vi "Linear Regression Code.vi"(7 "Ordered Pairs":T1, 10 "Number of Pairs":i32) -> (0 "Slope Angle":dbl, 3 "Intercept":dbl)   [LabVIEW 2012]
uses:
  <vilib>/Analysis/Matrix/Datatypes/RealMatrix.ctl
  <vilib>/Analysis/Matrix/NI_Matrix.lvlib
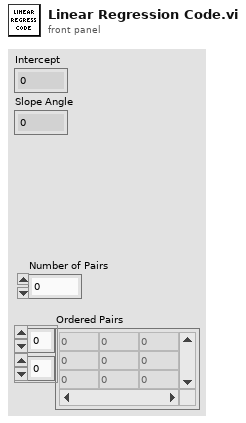
[diagram p1: front panel]
types:
  T1 = typedef "NI_Matrix.lvlib/RealMatrix.ctl" = dbl[][]
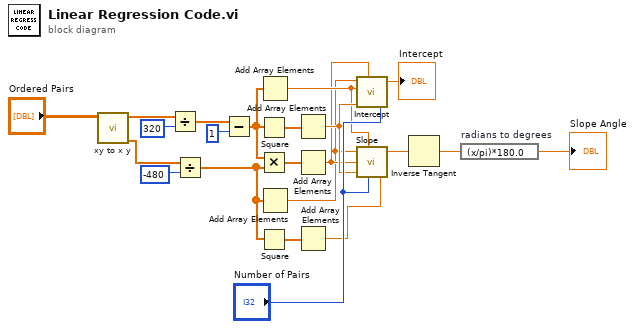
[diagram p0: block diagram]
diagram:
  n1 = call "xy to x y.vi"("Ordered Pairs"="Ordered Pairs") -> ("Y"=w1:dbl[], "X"=w2:dbl[])  [unwired: 9 in]
  n2 = Divide(x=w2, y=320) -> (x/y=w21:dbl[])
  n3 = Divide(x=w1, y=-480) -> (x/y=w15:dbl[])
  n4 = Subtract(x=w21, y=1) -> (x-y=w17:dbl[])
  n5 = Square(x=w17) -> (x^2=w16:dbl[])
  n6 = Multiply(x=w17, y=w15) -> (x*y=w18:dbl[])
  n7 = Square(x=w15) -> (x^2=w14:dbl[])
  n8 = Add Array Elements(numeric array=w17) -> (sum=w11:dbl)
  n9 = Add Array Elements(numeric array=w15) -> (sum=w9:dbl)
  n10 = Add Array Elements(numeric array=w16) -> (sum=w12:dbl)
  n11 = Add Array Elements(numeric array=w18) -> (sum=w10:dbl)
  n12 = Add Array Elements(numeric array=w14) -> (sum=w6:dbl)
  n13 = call "Intercept.vi"("Y"=w9, "X"=w11, "X2"=w12, "XY"=w10, "N"="Number of Pairs") -> ("Intercept"=→"Intercept":dbl)  [unwired: 2 in]
  n14 = call "Slope.vi"("Y"=w9, "X"=w11, "XY"=w10, "X2"=w12, "N"="Number of Pairs", "Y2"=w6) -> ("Slope"=w7:dbl)  [unwired: 1 in]
  n15 = Inverse Tangent(1:w7) -> (0:w8:dbl)
  n16 = expression code="(x/pi)*180.0" "radians to degrees"(w8) -> (→"Slope Angle":dbl)
